vi "Read.vi"(11 "MuxRoute Value in":refnum<class "MuxRoute Value.lvclass">) -> (2 "Muxes":cluster{"Mux Route":i32[]}[](array[cluster]))   [LabVIEW 2022 SP3, in "VideoMux.lvlib" / "MuxRoute Value.lvclass"]
uses:
  MuxRoute Value.lvclass
  MuxRoute Value.lvclass/MuxRoute Value.ctl
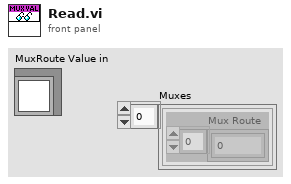
[diagram p1: front panel]
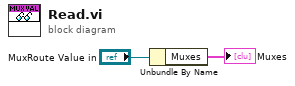
[diagram p0: block diagram]
diagram:
  n1 = Unbundle By Name("MuxRoute Value in") -> ("Muxes"=→"Muxes":cluster{"Mux Route":i32[]}[])
